vi "Remote Video still, with averaging.vi"(0 "Resolution":T1=1 items=["Low", "Med", "High", "Max."], 1 "Quality":u32=750 max=1000, 2 "Duration (s)":dbl=10.0 format="%#_13g", 3 "Averaging time (s) (from end)":dbl=1.0 format="%#_13g", 4 "Camera":T2="Travcam") -> (5 "Error out":errorcluster)   [LabVIEW 2015]
uses:
  Camera enum/Camera enum.ctl
  Camera enum/Camera resolution.ctl
  Globals/CamServer global.vi
panel:
  # "PN 27/08/15"
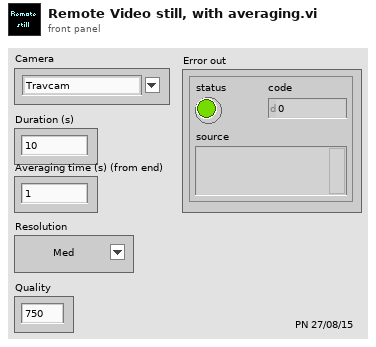
[diagram p1: front panel]
types:
  T1 = typedef "Camera resolution.ctl" = u8
  T2 = typedef "Camera enum.ctl" = string
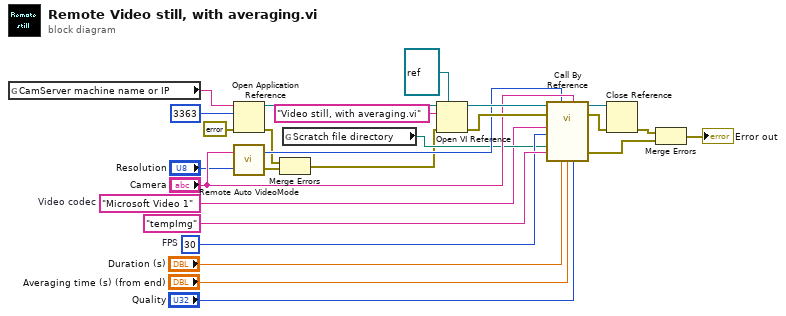
[diagram p0: block diagram]
diagram:
  w3 = "Microsoft Video 1"  # Video codec
  w11 = u32 30  # FPS
  n1 = global read "CamServer global.vi" "CamServer machine name or IP"() -> (w7:string)
  n2 = Open Application Reference(8:errorcluster {"status"=FALSE, "code"=0, "source"=""} ("error in (no error)"), 10:u16 3363 ("port"), 11:w7) -> (0:w6:errorcluster, 3:w24:refnum<vi>)  [unwired: 1 in]
  n3 = call "Remote Auto VideoMode.vi"("Resolution"="Resolution", "Camera"="Camera") -> ("Error out"=w5:errorcluster, "VideoMode"=w14:u32)
  n4 = Merge Errors(w6, w5) -> (w4:errorcluster)
  n5 = global read "CamServer global.vi" "Scratch file directory"() -> (w8:path)
  n6 = Open VI Reference(type specifier VI Refnum (for type only)=refnum<vi> refnum, application reference (local)=w24, vi path="Video still, with averaging.vi" ("machine name"), error in (no error)=w4) -> (vi reference=w22:refnum<vi>, error out=w23:errorcluster)  [unwired: 2 in]
  n7 = call-by-ref "?"(reference=w22, error in=w23, "Video codec"=w3, "VideoMode"=w14, "Interface name"="Camera", "FPS"=w11, "Image directory path"=w8, "Image name"="tempImg", "Duration (s)"="Duration (s)", "Averaging time (s) (from end)"="Averaging time (s) (from end)", "Quality"="Quality") -> (reference out=w20:refnum<vi>, error out=w19:errorcluster, "Error Out"=w18:errorcluster)  [unwired: 5 in, 1 out]
  n8 = Close Reference(reference=w20, error in (no error)=w19) -> (error out=w17:errorcluster)
  n9 = Merge Errors(w17, w18) -> (→"Error out":errorcluster)
